vi "fields Template Keys.vi"(7 "Display Name (\"\")":string, 8 "error in (no error)":errorcluster, 9 "Copy? (f)":bool, 10 "Edit? (f)":bool, 11 "Connection Refnum":T1) -> (0 "error out":errorcluster, 1 "Template Keys":T2, 3 "Connection Refnum":T1)   [LabVIEW 2011]
uses:
  ITK EXT/utils/keyedarr.llb/Keyed Array.ctl
  Summitek EXT/ODBC/SQL Controls/Connection Refnum.ctl
  server/database/Fields/Field Order By.ctl
  ITK EXT/utils/strutil.llb/Case Matching.ctl
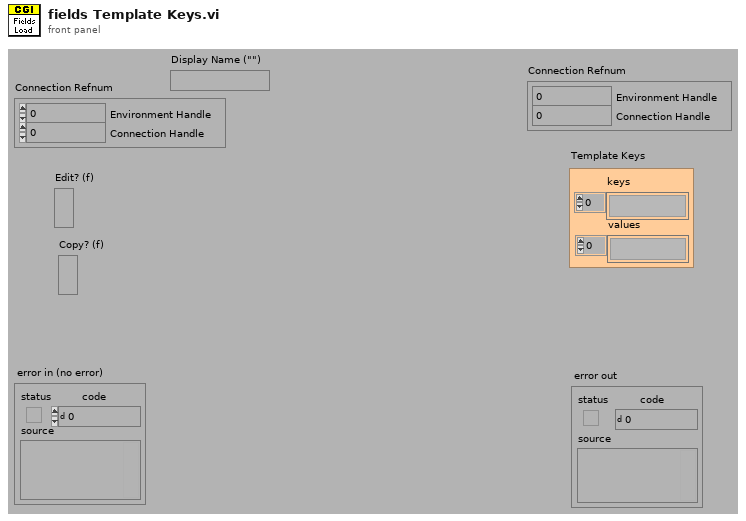
[diagram p1: front panel]
types:
  T1 = typedef "Connection Refnum.ctl" = cluster{"Environment Handle":i32, "Connection Handle":i32}
  T2 = typedef "Keyed Array.ctl" = cluster{"keys":string[], "values":string[]}
  T3 = typedef "Field Order By.ctl" = enum32{"sxSequenceId", "sxFieldId", "sDisplayName", "sValue", "fSetAtTest", "fRequired", "nNextItem"}
  T4 = typedef "Field Record.ctl" = cluster{"ixField":i32, "iSequenceOrder":i32, "sxFieldId":string, "sxSequenceId":string, "sDisplayName":string, "sValue":string, "sUnits":string, "nDataType":T5, "nNextItem":T6, "fSystem":bool, "fSystemValue":bool, "fRequired":bool, "fSetAtTest":bool, "fTestField":bool, "fDeleted":bool, "fIndexed":bool, "fFreeList":bool}
  T5 = typedef "Field DataTypes.ctl" = enum32{"text", "numeric", "list", "timestamp", "boolean"}
  T6 = typedef "Field NextItem.ctl" = enum32{"Reset", "Retain", "Auto-Increment"}
  T7 = typedef "Case Matching.ctl" = enum16{"a != A", "a == A", "system"}
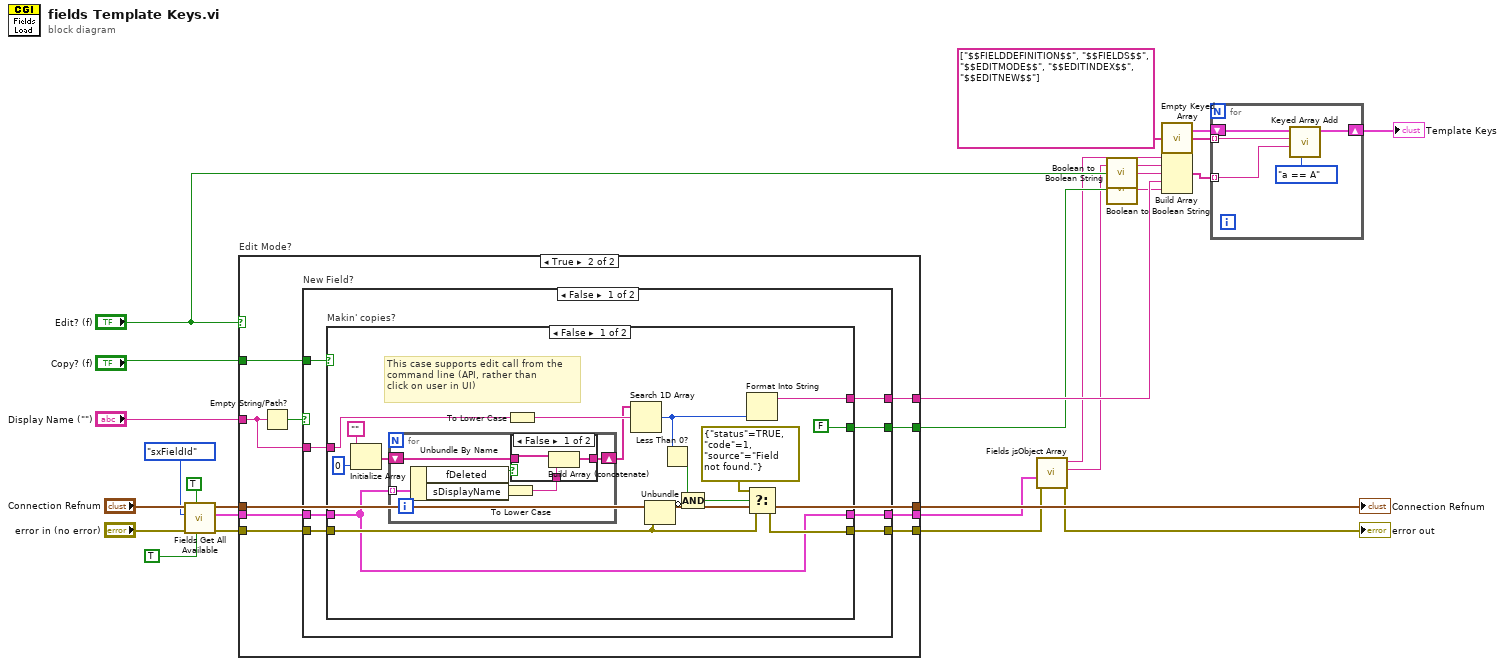
[diagram p0: block diagram]
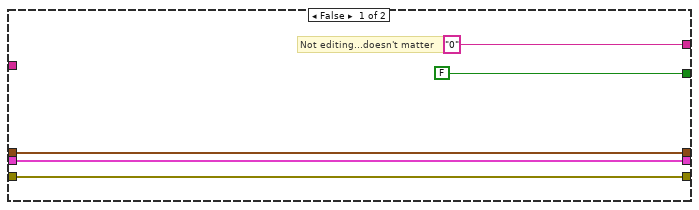
[diagram p2: hidden frame]
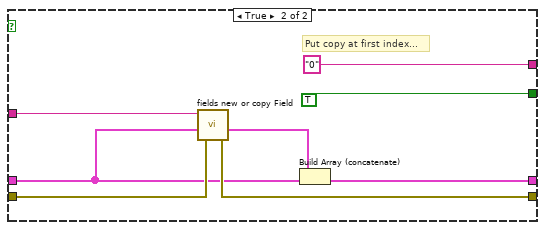
[diagram p4: hidden frame]
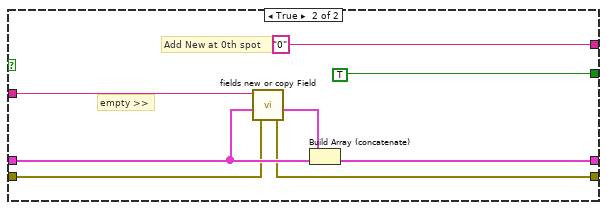
[diagram p5: hidden frame]
diagram:
  n1 = call "Fields Get All Available.vi"("Combine All? (f)"=TRUE, "Include Deleted? (F)"=TRUE, "error in (no error)"="error in (no error)", "Sort by (sxSequenceId)"=Field_Order_By."sxFieldId" ("Sort by (Sequence_ID)"), "Connection Refnum"="Connection Refnum") -> ("error out"=w19:errorcluster, "System or ALL Combined Fields"=w2:T4[], "Connection Refnum"=w14:T1)  [unwired: 1 in, 3 out]
  n2 = case "Edit Mode?" shown="True" "Edit? (f)" {
    tunnel: w2 -> [w27 w40]
    tunnel: w19 -> [w30 w38]
    tunnel: [w30 w37] -> w8
    tunnel: ["0" w36] -> w17
    tunnel: [w27 w35] -> w7
    tunnel: "Display Name (\"\")" -> [_ w34]
    tunnel: w14 -> [w28 w32]
    tunnel: [w28 w32] -> w13
    tunnel: "Copy? (f)" -> [_ w33]
    tunnel: [FALSE w31] -> w10
    frame False {
      # "Not editing...doesn't matter"
    }
    frame True {
      n3 = Empty String/Path?(string/path=w34) -> (empty?=w39:bool)
      n4 = case "New Field?" shown="False" w39 {
        tunnel: w40 -> [w45 w88]
        tunnel: w38 -> [w46 w86]
        tunnel: [w47 w85] -> w37
        tunnel: [w42 w90] -> w35
        tunnel: [w48 "0"] -> w36
        tunnel: w34 -> [w44 w83]
        tunnel: w33 -> [w43 _]
        tunnel: [w41 TRUE] -> w31
        frame False {
          n5 = case "Makin' copies?" shown="False" w43 {
            tunnel: [w62 "0"] -> w48
            tunnel: [w61 w78] -> w47
            tunnel: w46 -> [w60 w79]
            tunnel: w45 -> [w54 w77]
            tunnel: w44 -> [w55 w75]
            tunnel: [w54 w81] -> w42
            tunnel: [FALSE TRUE] -> w41
            frame False {
              # "This case supports edit call from the\ncommand line (API, rather than\nclick on user in UI)"
              n6 = Initialize Array("", 0 ("dimension size")) -> (w52:string[])
              n7 = for {
                tunnel: w54 -> [w70] mode=indexing
                shift-right: [w66] -> w49
                shift-left: w52 -> [w67]
                n8 = Unbundle By Name(w70) -> ("fDeleted"=w68:bool, "sDisplayName"=w69:string)
                n9 = To Lower Case(string=w69) -> (all lower case string=w65:string)
                n10 = case shown="False" w68 {
                  tunnel: w67 -> [w71 w74]
                  tunnel: [w73 w74] -> w66
                  tunnel: w65 -> [w72 _]
                  frame False {
                    n11 = Build Array (concatenate)(w71, w72) -> (w73:string[])
                  }
                  frame True {
                  }
                }
              }
              n12 = To Lower Case(string=w55) -> (all lower case string=w64:string)
              n13 = Search 1D Array(1D array=w49, element=w64) -> (index of element=w63:i32)  [unwired: 1 out]
              n14 = Unbundle(w60) -> ("status"=w59:bool)  [unwired: 2 out]
              n15 = Less Than 0?(x=w63) -> (x < 0?=w58:bool)
              n16 = Compound Arithmetic op=AND(w58, invert w59) -> (w57:bool)
              n17 = Format Into String(w63) -> (resulting string=w62:string)  [unwired: 3 in, 1 out]
              n18 = Select(t=errorcluster {"status"=TRUE, "code"=1, "source"="Field not found."}, s=w57, f=w60) -> (s? t:f=w61:errorcluster)
            }
            frame True {
              # "Put copy at first index..."
              n19 = call "fields new or copy Field.vi"("error in (no error)"=w79, "All Fields (empty)"=w77, "Copy Existing? (\"\": new field)"=w75) -> ("error out"=w78:errorcluster, "New Field Record"=w80:T4)  [unwired: 1 in, 2 out]
              n20 = Build Array (concatenate)(w80, w77) -> (w81:T4[])
            }
          }
        }
        frame True {
          # "empty >>"
          # "Add New at 0th spot"
          n21 = call "fields new or copy Field.vi"("error in (no error)"=w86, "All Fields (empty)"=w88, "Copy Existing? (\"\": new field)"=w83) -> ("error out"=w85:errorcluster, "New Field Record"=w87:T4)  [unwired: 1 in, 2 out]
          n22 = Build Array (concatenate)(w87, w88) -> (w90:T4[])
        }
      }
    }
  }
  "Connection Refnum" <- w13
  n23 = call "Fields jsObject Array.vi"("error in (no error)"=w8, "FIELDS (none)"=w7) -> ("error out"=→"error out":errorcluster, "Fields jsObject Array"=w4:string, "Field jsObject Definition"=w5:string)  [unwired: 2 in, 5 out]
  n24 = call "Boolean to Boolean String.vi"("Boolean"="Edit? (f)") -> ("Boolean string"=w16:string)  [unwired: 1 in]
  n25 = call "Boolean to Boolean String.vi"("Boolean"=w10) -> ("Boolean string"=w11:string)  [unwired: 1 in]
  n26 = call "Empty Keyed Array.vi"() -> ("empty keyed array"=w23:T2)  [unwired: 3 out]
  n27 = Build Array(w5, w4, w16, w17, w11) -> (w22:string[])
  n28 = for {
    shift-right: [w92] -> w21
    shift-left: w23 -> [w94]
    tunnel: string[] ["$$FIELDDEFINITION$$", "$$FIELDS$$", "$$EDITMODE$$", "$$EDITINDEX$$", "$$EDITNEW$$"] -> [w93] mode=indexing
    tunnel: w22 -> [w91] mode=indexing
    n29 = call "Keyed Array Add.vi"("case matching (sensitive)"=Case_Matching."a == A", "value"=w91, "key"=w93, "array in"=w94) -> ("array out"=w92:T2)  [unwired: 3 out]
  }
  "Template Keys" <- w21
